vi "vision_webcam_V2_external_use.vi"(11 "dup Message Queue 2":refnum<queue>) -> ()   [LabVIEW 2017]
uses:
  UI Error Handlers/support/Message Queue/Message Cluster.ctl
  <vilib>/userdefined/High Color/IMAQdx.ctl
  Control 2.ctl
  <vilib>/vision/Image Controls.llb/IMAQ Image.ctl
  Globals/Global - All RT Loop Stop.vi
  Globals/Global - Configuration Options.vi
  <vilib>/vision/driver/NI_Vision_Acquisition_Software.lvlib
  UI Error Handlers/support/Message Queue/Message Queue.lvlib
panel:
  out "appended path":path
  out "Webcam":T1(plugin-control)
  out "concatenated string 4":string
  out "error out":errorcluster
  out "x-y":u32
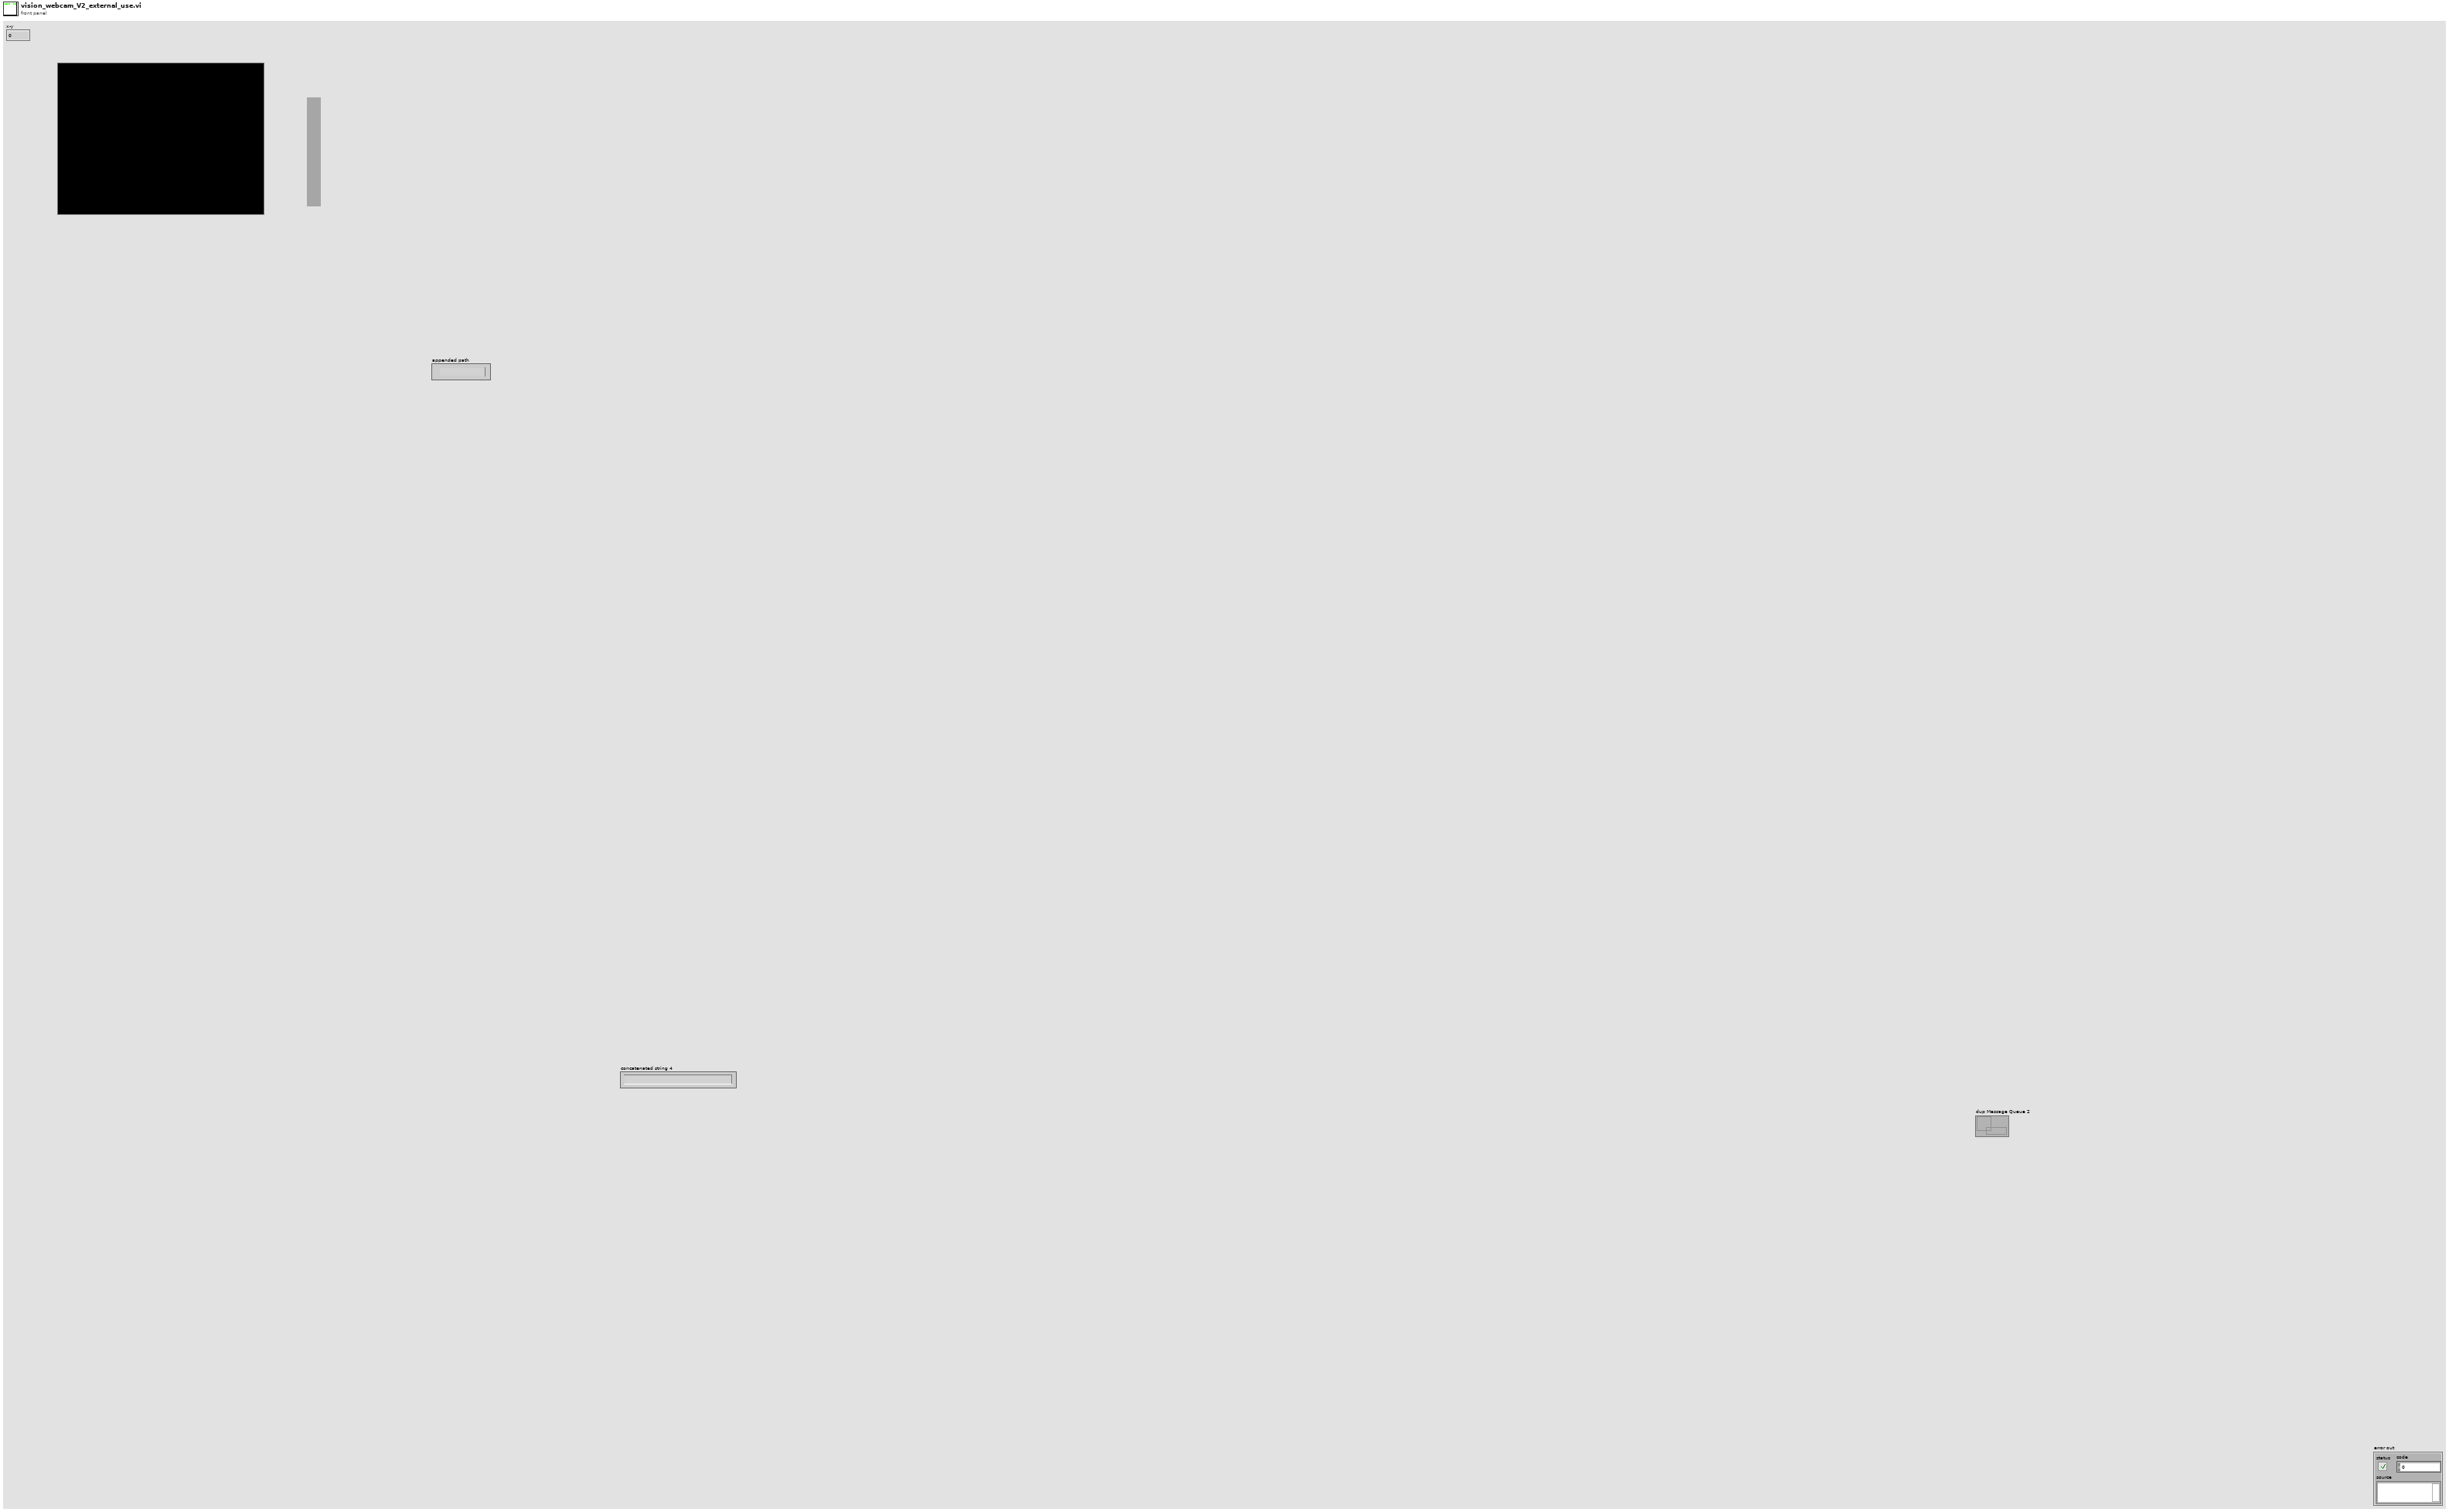
[diagram p1: front panel]
types:
  T1 = typedef "IMAQ Image.ctl" = refnum<image>
  T2 = typedef "Control 2.ctl" = T1[]
  T3 = typedef "IMAQdx.ctl" = refnum<k21>
  T4 = typedef "Image Type" = u32
  T5 = cluster{"Tool data":cluster{"Number of teeth":sgl}, "Cutting data":cluster{"rpm":sgl}, "Limits":cluster{"Magnitude threshold":sgl, "Tolerance":sgl}, "G1 status":cluster{"G1 trigger":bool}}
  T6 = typedef "IMAQ AVI2 Refnum.ctl" = refnum<k20>
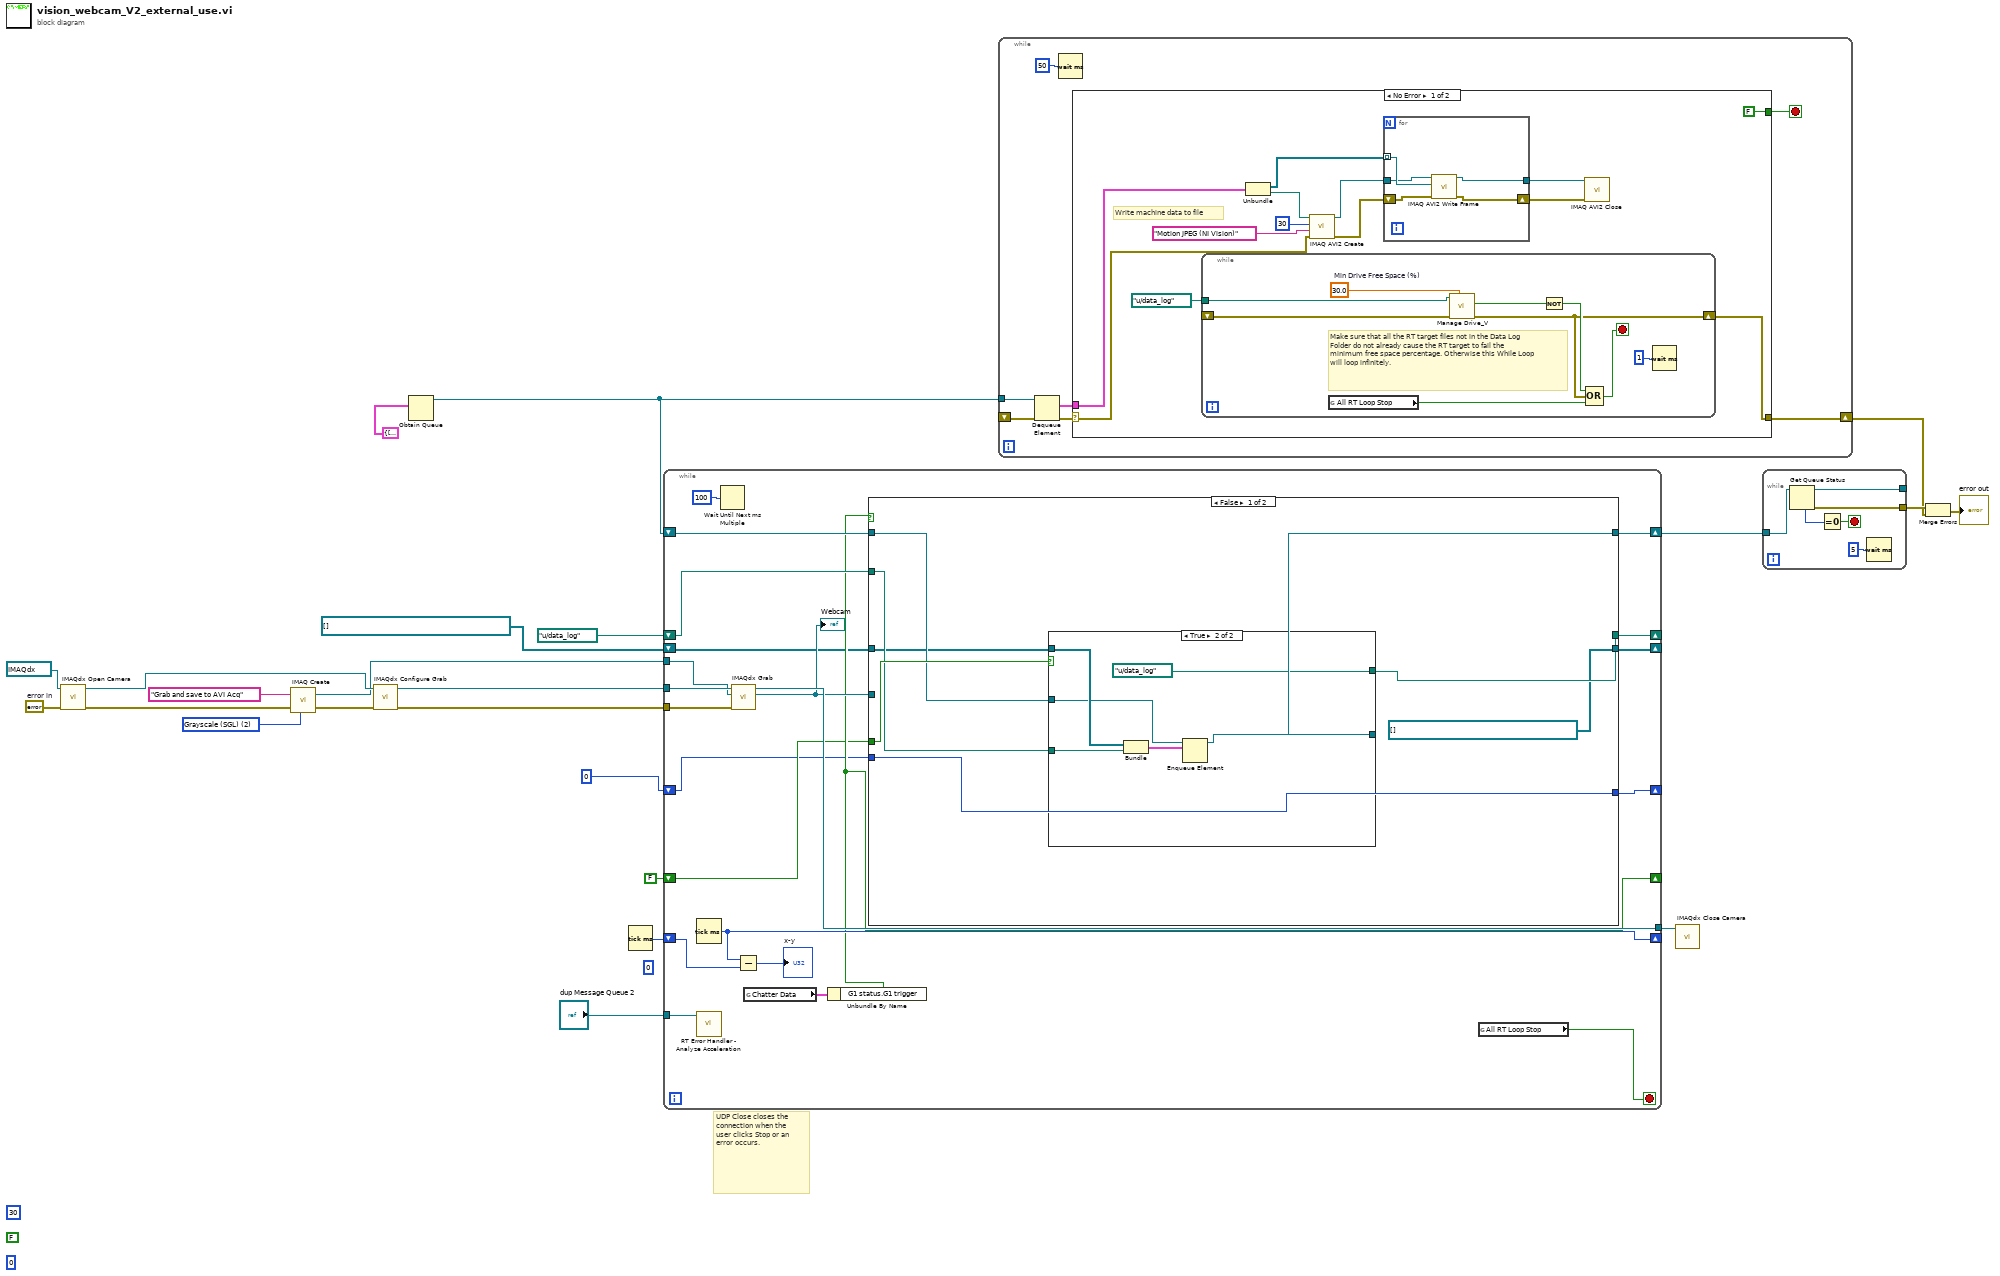
[diagram p0: block diagram]
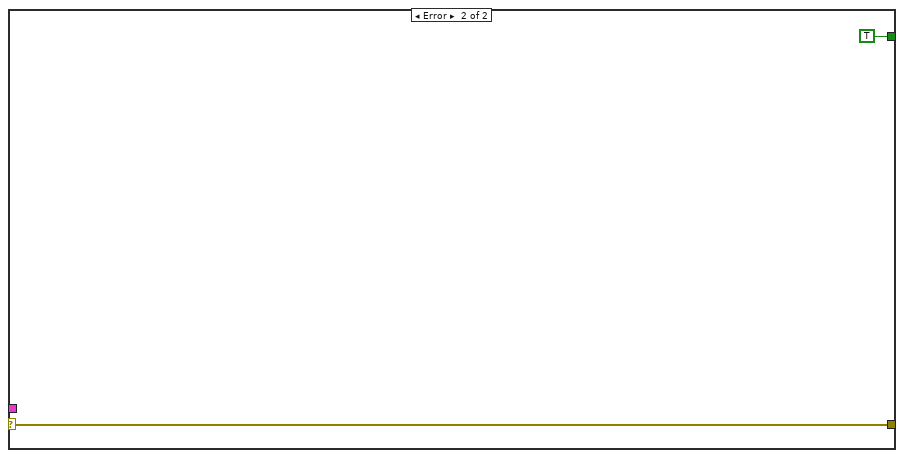
[diagram p2: hidden frame]
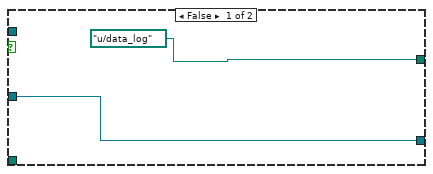
[diagram p3: hidden frame]
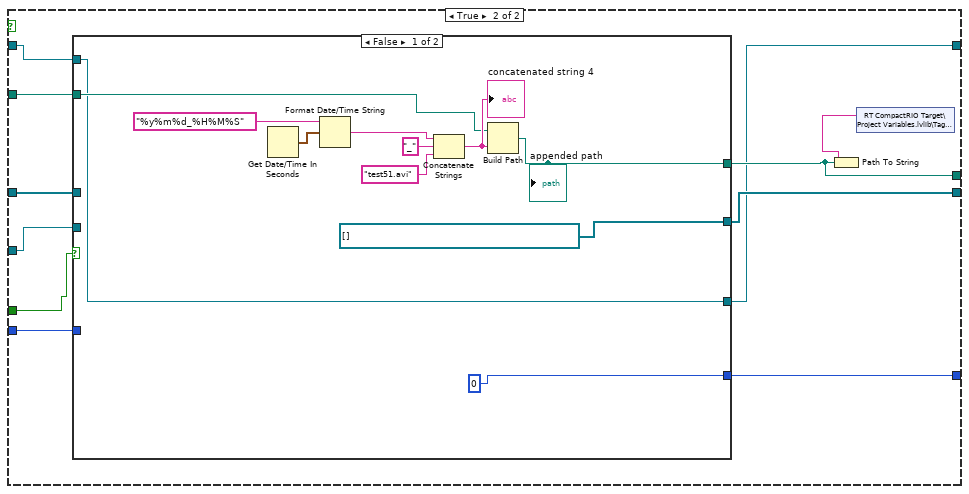
[diagram p4: hidden frame]
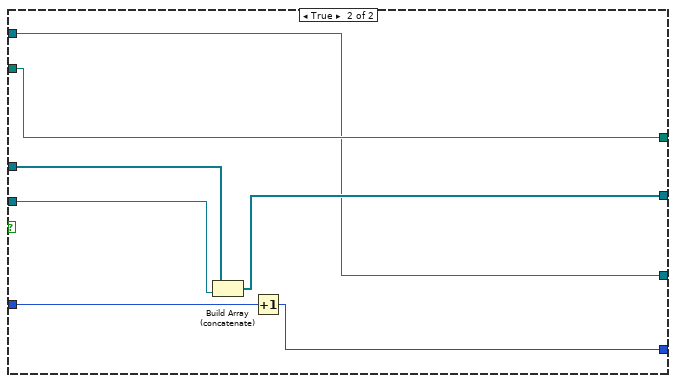
[diagram p5: hidden frame]
diagram:
  (unwired) 0
  w13 = T4 2 items=["Grayscale (U8)", "Grayscale (I16)", "Grayscale (SGL)", "Complex (CSG)", "RGB (U32)", "HSL (U32)", "RGB (U64)", "Grayscale (U16)"] ("Image Type")
  (unwired) u32 30 ("Frames Per Second")
  w14 = errorcluster {"status"=FALSE, "code"=0, "source"=""}  # error in
  (unwired) i16 0 ("A(I16) 11")
  (unwired) FALSE
  # "UDP Close closes the connection when the user clicks Stop or an error occurs."
  n1 = call <vilib>:"IMAQdx Open Camera.vi"("error in"=w14, "Session In"=T3 "cam1") -> ("error out"=w12:errorcluster, "Session Out"=w16:T3)  [unwired: 8 in]
  n2 = call "IMAQ Create"("Image Name"="Grab and save to AVI Acq", "Image Type"=w13, "error in (no error)"=w12) -> ("New Image"=w9:T1, "error out"=w8:errorcluster)  [unwired: 2 in]
  n3 = call <vilib>:"IMAQdx Configure Grab.vi"("error in"=w8, "Session In"=w16) -> ("error out"=w7:errorcluster, "Session Out"=w10:T3)  [unwired: 8 in]
  n4 = Obtain Queue(element data type=cluster{T2, "appended path 2":path} {[], "appended path 2"=path ""}) -> (queue out=w21:refnum<queue>)  [unwired: 4 in, 2 out]
  n5 = Tick Count (ms)() -> (millisecond timer value=w17:u32)
  n6 = while {
    shift-right: [w44] -> w23
    shift-left: w21 -> [w45]
    tunnel: "dup Message Queue 2" -> [w43]
    shift-right: [w39] -> _
    shift-left: w17 -> [w40]
    tunnel: w10 -> [w38]
    tunnel: w9 -> [w37]
    tunnel: w7 -> [w36]
    tunnel: [w35] -> w6
    shift-right: [w30] -> _
    shift-left: path "u:/data_log" ("AVI Path") -> [w31]
    shift-right: [w29] -> _
    shift-left: FALSE ("G1 trigger") -> [w28]
    shift-right: [w27] -> _
    shift-left: T2 [] -> [w24]
    shift-right: [w25] -> _
    shift-left: 0 -> [w26]
    stop <- w33 stop-if-true
    n7 = Tick Count (ms)() -> (millisecond timer value=w39:u32)
    n8 = call "RT Error Handler - Analyze Acceleration.vi"("Message Queue"=w43) -> ()  [unwired: 10 in, 1 out]
    n9 = Wait Until Next ms Multiple(millisecond multiple=u32 100) -> ()  [unwired: 1 out]
    n10 = call <vilib>:"IMAQdx Grab.vi"("error in"=w36, "Image In"=w37, "Session In"=w38) -> ("Image Out"=w32:T1, "Session Out"=w35:T3)  [unwired: 5 in, 2 out]
    "Webcam" <- w32
    n11 = Subtract(x=w39, y=w40) -> (x-y=→"x-y":u32)
    n12 = global read "Global - Configuration Options.vi" "Chatter Data"() -> (w42:T5)
    n13 = Unbundle By Name(w42) -> ("G1 status.G1 trigger"=w29:bool)
    n14 = case shown="False" w29 {
      tunnel: w45 -> [w51 w63]
      tunnel: [w48 w62] -> w44
      tunnel: w32 -> [_ w72]
      tunnel: w31 -> [w50 w70]
      tunnel: [w53 w69] -> w30
      tunnel: w28 -> [w52 w68]
      tunnel: [T2 [] w67] -> w27
      tunnel: w26 -> [w47 w66]
      tunnel: [w47 w65] -> w25
      tunnel: w24 -> [w49 w64]
      frame False {
        n15 = case shown="True" w52 {
          tunnel: [path "u:/data_log" ("AVI Path") path "u:/data_log" ("AVI Path")] -> w53
          tunnel: w51 -> [w54 w58]
          tunnel: w50 -> [_ w60]
          tunnel: w49 -> [_ w59]
          tunnel: [w54 w56] -> w48
          frame False {
          }
          frame True {
            n16 = Bundle(w59, "AVI Path"=w60) -> (w57:cluster{T2, "AVI Path":path})  [unwired: 1 in]
            n17 = Enqueue Element(queue=w58, element=w57) -> (queue out=w56:refnum<queue>)  [unwired: 2 in, 2 out]
          }
        }
      }
      frame True {
        n18 = case shown="False" w68 {
          tunnel: w72 -> [_ w89]
          tunnel: w63 -> [w73 w84]
          tunnel: [w77 w90] -> w69
          tunnel: w70 -> [w76 w90]
          tunnel: [T2 [] w85] -> w67
          tunnel: w66 -> [_ w88]
          tunnel: [0 w87] -> w65
          tunnel: w64 -> [_ w86]
          tunnel: [w73 w84] -> w62
          frame False {
            n19 = Get Date/Time In Seconds() -> (seconds since 1Jan1904=w81:timestamp)
            n20 = Format Date/Time String(time format string (%c)="%y%m%d_%H%M%S", seconds (now)=w81) -> (date/time string=w82:string)  [unwired: 1 out]
            n21 = Concatenate Strings(w82, "_" ("string"), "test51.avi" ("name or relative path")) -> (w83:string)
            "concatenated string 4" <- w83
            n22 = Build Path(base path=w76, name or relative path=w83) -> (appended path=w77:path)
            "appended path" <- w77
          }
          frame True {
            n23 = Build Array (concatenate)(w86, w89) -> (w85:T2)
            n24 = Increment(x=w88) -> (x+1=w87:i32)
          }
        }
        n25 = Path To String(path=w69) -> (string=w71:string)
        n26 = shared-variable "RT CompactRIO Target\\Project Variables.lvlib\\Tag Video"(w71) -> ()  [unwired: 1 in, 1 out]
      }
    }
    n27 = global read "Global - All RT Loop Stop.vi" "All RT Loop Stop"() -> (w33:bool)
  }
  n28 = while {
    tunnel: w21 -> [w97]
    shift-right: [w93] -> w20
    shift-left: _ -> [w96]
    stop <- w94 stop-if-true
    n29 = Dequeue Element(queue=w97, error in (no error)=w96) -> (element=w92:cluster{T2, "appended path 2":path}, error out=w95:errorcluster)  [unwired: 1 in, 2 out]
    n30 = Wait (ms)(milliseconds to wait=u32 50) -> ()  [unwired: 1 out]
    n31 = case shown="No Error" w95 {
      selector: w95 -> [w98 w125]
      tunnel: [FALSE TRUE] -> w94
      tunnel: [w108 w125] -> w93
      tunnel: w92 -> [w107 _]
      frame No Error {
        # "Write machine data to file"
        n32 = while {
          shift-right: [w119] -> w108
          shift-left: _ -> [w120]
          tunnel: path "u:/data_log" ("AVI Path") -> [w117]
          stop <- w124 stop-if-true
          w118 = 30.0  # Min Drive Free Space (%)
          # "Make sure that all the RT target files not in the Data Log Folder do not already cause the RT target to fail the minimum free space percentage. Otherwise this While Loop will loop infinitely."
          n33 = global read "Global - All RT Loop Stop.vi" "All RT Loop Stop"() -> (w121:bool)
          n34 = call "Manage Drive_V.vi"("Min Drive Free Space (%)"=w118, "error in"=w120, "Data Folder"=w117) -> ("error out"=w119:errorcluster, "Drive Space Below Limit"=w116:bool)  [unwired: 6 in, 1 out]
          n35 = Not(x=w116) -> (.not. x?=w123:bool)
          n36 = Compound Arithmetic op=OR(w123, w119, w121) -> (w124:bool)
          n37 = Wait (ms)(milliseconds to wait=u32 1) -> ()  [unwired: 1 out]
        }
        n38 = Unbundle(w107) -> (w106:T2, "appended path 2"=w103:path)
        n39 = call "IMAQ AVI2 Create"("error in (no error)"=w98, "Codec"="Motion JPEG (NI Vision)", "Frames Per Second"=u32 30, "AVI Path"=w103) -> ("error out"=w99:errorcluster, "AVI Refnum"=w102:T6)  [unwired: 6 in]
        n40 = for {
          tunnel: w106 -> [w115] mode=indexing
          tunnel: w102 -> [w114]
          tunnel: [w113] -> w101
          shift-right: [w112] -> w100
          shift-left: w99 -> [w111]
          n41 = call "IMAQ AVI2 Write Frame"("error in (no error)"=w111, "Image"=w115, "AVI Refnum"=w114) -> ("error out"=w112:errorcluster, "AVI Refnum (duplicate)"=w113:T6)  [unwired: 6 in, 1 out]
        }
        n42 = call "IMAQ AVI2 Close"("error in (no error)"=w100, "AVI Refnum"=w101) -> ()  [unwired: 9 in, 1 out]
      }
      frame Error {
      }
    }
  }
  n43 = call <vilib>:"IMAQdx Close Camera.vi"("Session In"=w6) -> ()  [unwired: 10 in, 1 out]
  n44 = while {
    tunnel: [w131] -> w22
    tunnel: [w129] -> _
    tunnel: w23 -> [w127]
    stop <- w130 stop-if-true
    n45 = Get Queue Status(queue=w127) -> (queue out=w129:refnum<queue>, error out=w131:errorcluster, # elements in queue=w128:i32)  [unwired: 2 in, 5 out]
    n46 = Equal To 0?(x=w128) -> (x = 0?=w130:bool)
    n47 = Wait (ms)(milliseconds to wait=u32 5) -> ()  [unwired: 1 out]
  }
  n48 = Merge Errors(w22, w20) -> (→"error out":errorcluster)
